vi "Calling VI - Friend of Class A.vi"   [LabVIEW 2023]
doc: "This VI is not a member of any LabVIEW class but Class A designates it as a friend."
uses:
  Class A/Class A.lvclass
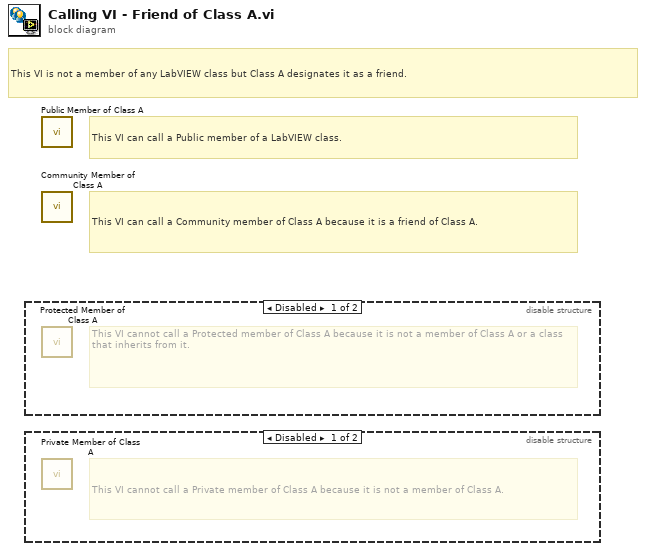
[diagram p0: block diagram]
diagram:
  # "This VI can call a Community member of Class A because it is a friend of Class A."
  # "This VI can call a Public member of a LabVIEW class."
  # "This VI is not a member of any LabVIEW class but Class A designates it as a friend."
  n1 = disable-structure shown="Disabled" {
    frame Disabled {
      # "This VI cannot call a Protected member of Class A because it is not a member of Class A or a class that inherits from it."
      n2 = call "Protected Member of Class A.vi"() -> ()  [unwired: 12 in]
    }
    frame Enabled {
    }
  }
  n3 = disable-structure shown="Disabled" {
    frame Disabled {
      # "This VI cannot call a Private member of Class A because it is not a member of Class A."
      n4 = call "Private Member of Class A.vi"() -> ()  [unwired: 12 in]
    }
    frame Enabled {
    }
  }
  n5 = call "Public Member of Class A.vi"() -> ()  [unwired: 12 in]
  n6 = call "Community Member of Class A.vi"() -> ()  [unwired: 12 in]
